vi "显示曲线1.vi"(2 "力觉参数":T1 {"下限" format="%.1f"; "上限" format="%.1f"; "系数" format="%.3f"}, 3 "力数组":sgl[](array[numeric]) format="%.2f") -> (0 "力值":sgl format="%.3f", 1 "曲线":cluster{"值":sgl, "上限":sgl, "下限":sgl})   [LabVIEW 2018]
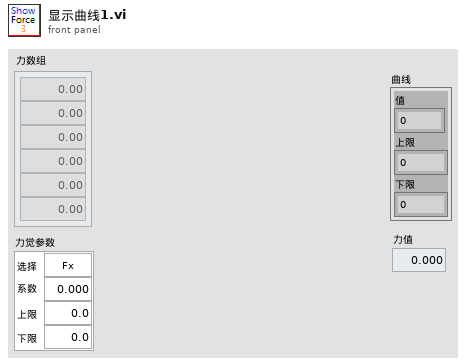
[diagram p1: front panel]
types:
  T1 = cluster{"选择":enum16{"Fx", "Fy", "Fz", "Mx", "My", "Mz"}, "系数":sgl, "上限":sgl, "下限":sgl}
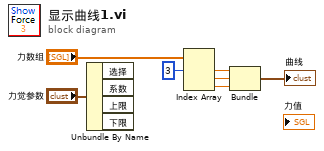
[diagram p0: block diagram]
diagram:
  n1 = Unbundle By Name("力觉参数") -> ()  [unwired: 4 out]
  n2 = Index Array(array="力数组", index #1=3 ("索引")) -> (element #1=w4:sgl, element #2=w3:sgl, element #3=w2:sgl)  [unwired: 2 in]
  n3 = Bundle("数值"=w4, "数值"=w3, "数值"=w2) -> (→"曲线":cluster{"数值":sgl, "数值":sgl, "数值":sgl})  [unwired: 1 in]
